vi "Init.vi"(8 "error in (no error)":errorcluster, 9 "permission":T1, 10 "name":string, 11 "Person in":refnum<class "Person.lvclass">) -> (0 "error out":errorcluster, 3 "Person out":refnum<class "Person.lvclass">)   [LabVIEW 2014, in "Person.lvclass"]
uses:
  Person.lvclass
  DEF-Permission.ctl
  Person.lvclass/Person.ctl
  ResetPermission.vi
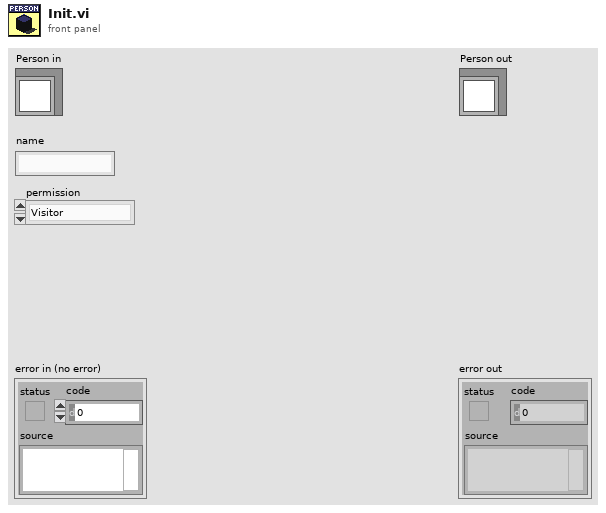
[diagram p1: front panel]
types:
  T1 = typedef "Person.lvclass/DEF-Permission.ctl" = enum16{"Visitor", "User", "Admin"}
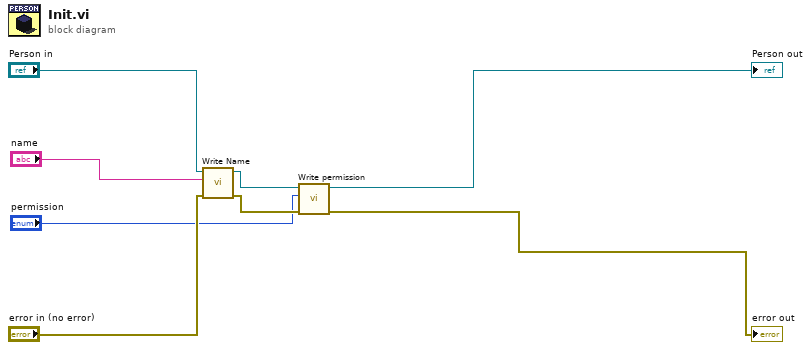
[diagram p0: block diagram]
diagram:
  n1 = call "Write Name.vi"("error in (no error)"="error in (no error)", "Name"="name", "Person in"="Person in") -> ("error out"=w4:errorcluster, "Person out"=w7:refnum<class "Person.lvclass">)  [unwired: 7 in]
  n2 = call "Write permission.vi"("error in (no error)"=w4, "permission"="permission", "Person in"=w7) -> ("error out"=→"error out":errorcluster, "Person out"=→"Person out":refnum<class "Person.lvclass">)  [unwired: 7 in]
